vi "Example - Send Client Message.vi"() -> ()   [LabVIEW 2020]
uses:
  <vilib>/ADAS Record/Utilities/TypeDefs/ADAS gRPC/DataStreamGrpc Message.ctl
  <vilib>/ADAS Record/Utilities/ADAS Utilities.lvlib
  <vilib>/DatastreamGrpc/DatastreamGrpc.lvlib
panel:
  in  "Stop":bool
  in  "SEND":bool
  out "error out":errorcluster
  in  "Tab Control":enum32{"Raw JSON", "messageName and Details"}(tab)
  in  "JSON string":string
  in  "messageName":string="Reconfigure"
  in  "details":string="{\"Config Path\":\"C:\\\\Users\\\\Public\\\\Documents\\\\National Instruments\\\\ADAS\\\\Config\\\\test_configB.json\",\"Engine History Length\":1}"
  out "Console Topic Response":string
  in  "timeout (ms)":u32=2000
  in  "Target Topic":T1(ring)
  # "Pre-formatted Reconfigure Details JSON"
  # "{\"Config Path\":\"C:\\\\Users\\\\Public\\\\Documents\\\\National Instruments\\\\ADAS\\\\Config\\\\test_configB.json\",\"Engine History Length\":1}"
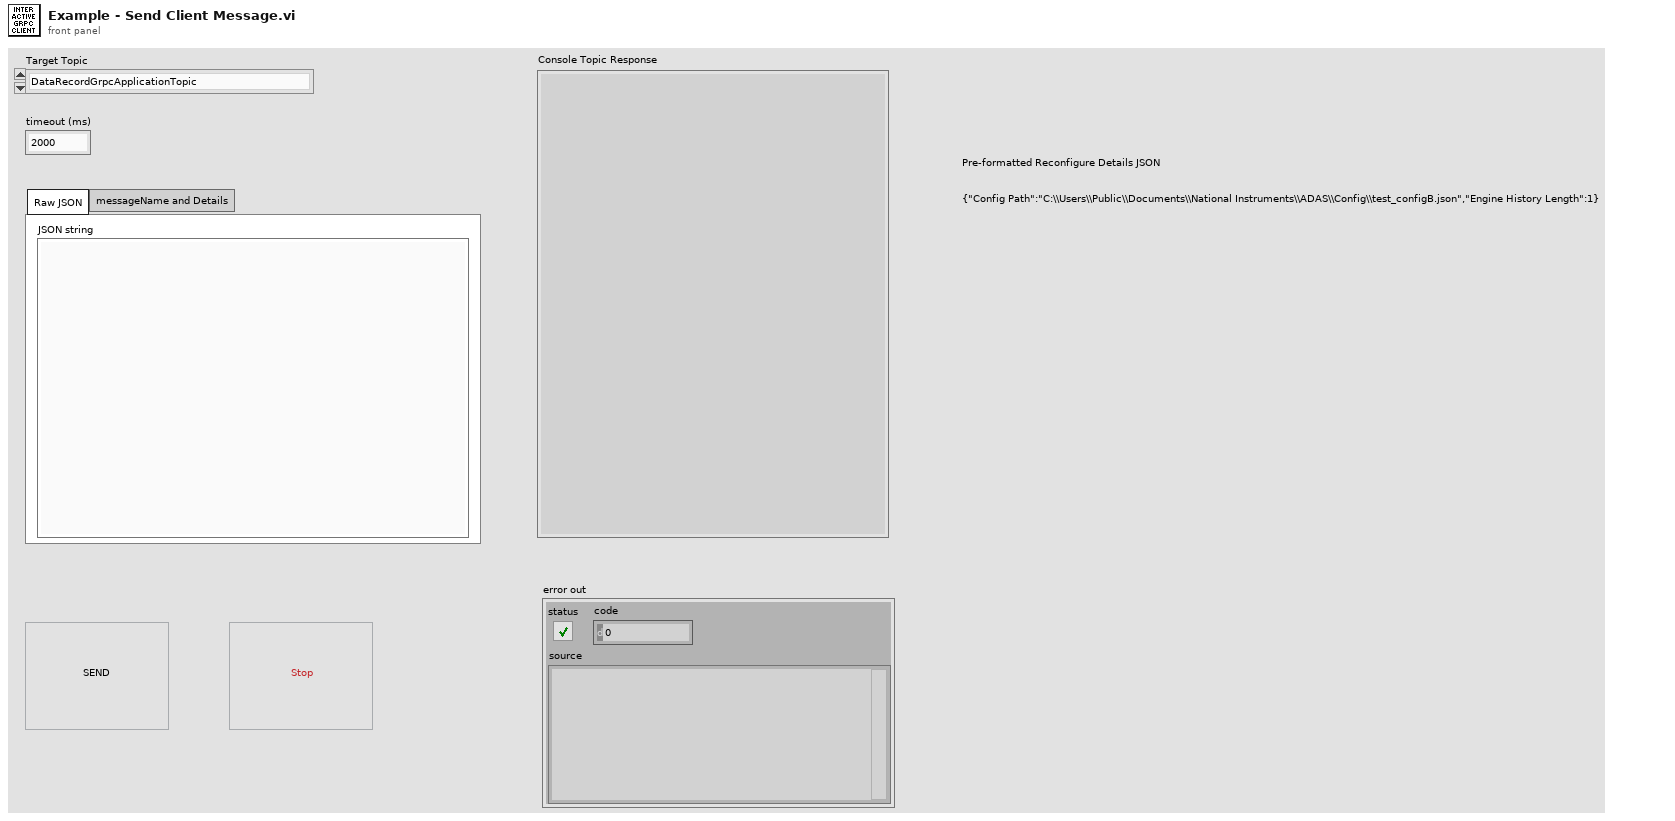
[diagram p1: front panel]
types:
  T1 = enum16{"DataRecordGrpcApplicationTopic", "DataRecordGrpcPluginTopic"}
  T2 = typedef "ADAS Utilities.lvlib/DataStreamGrpc Message.ctl" = cluster{"messageName":string, "details":string}
  T3 = typedef "DatastreamGrpc.lvlib/ClientRef.ctl" = cluster{"id":u64}
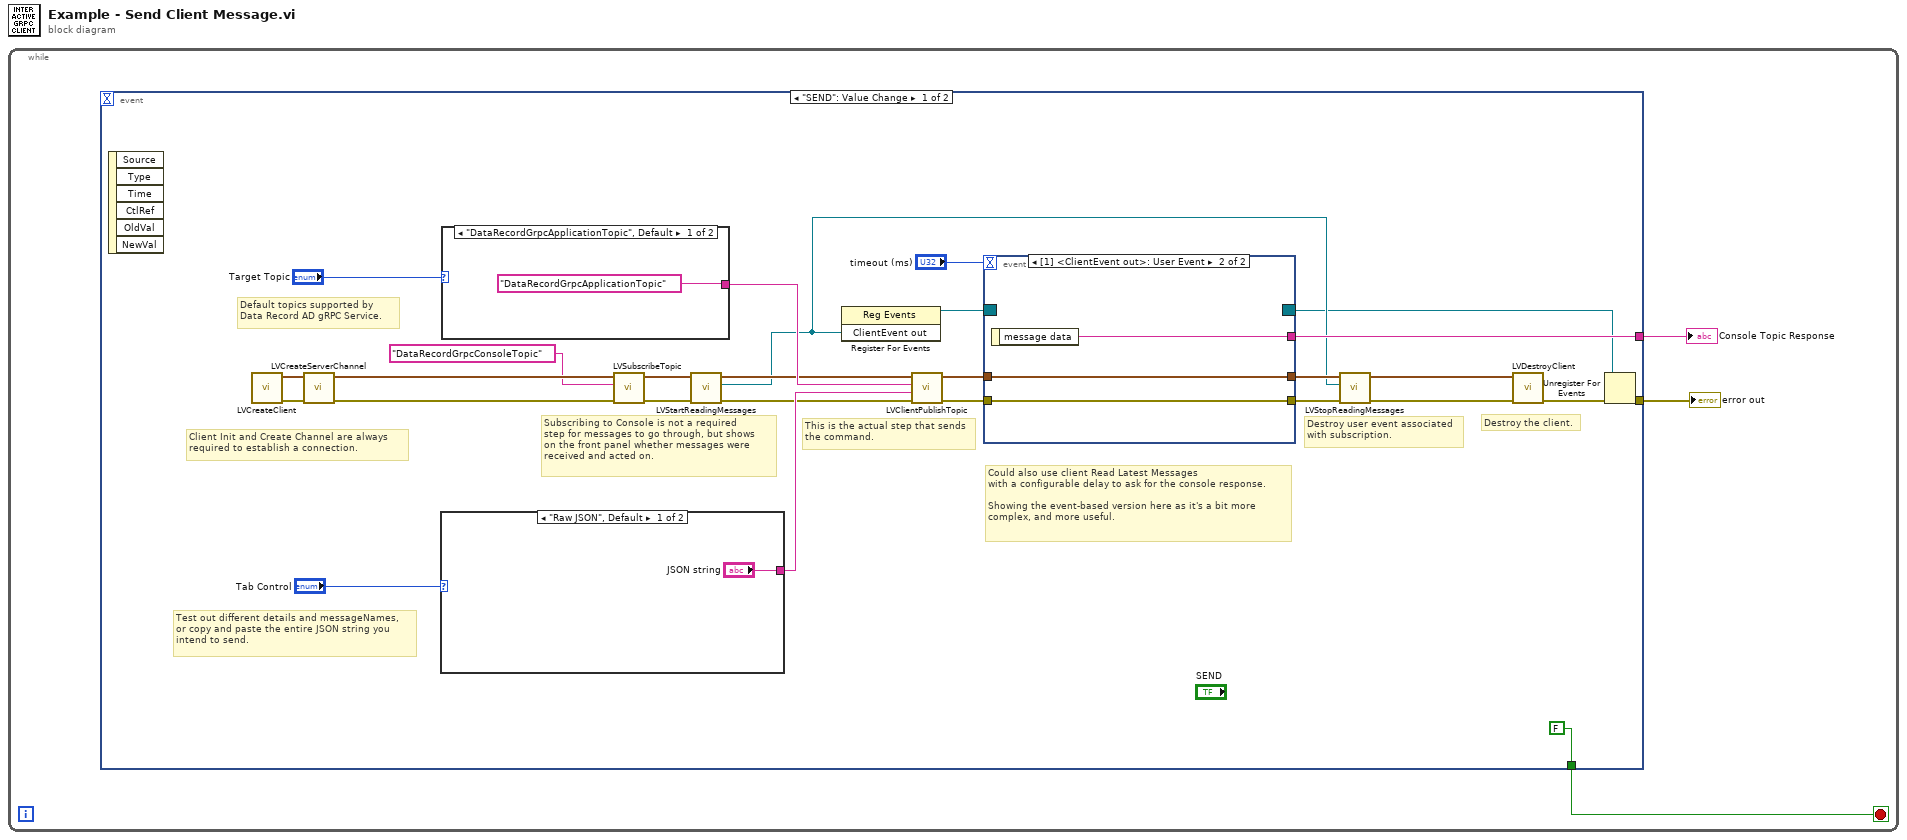
[diagram p0: block diagram]
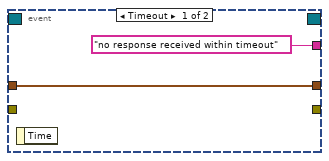
[diagram p2: hidden frame]
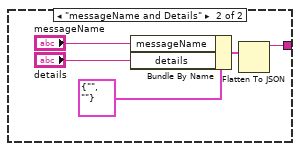
[diagram p3: hidden frame]
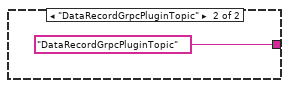
[diagram p4: hidden frame]
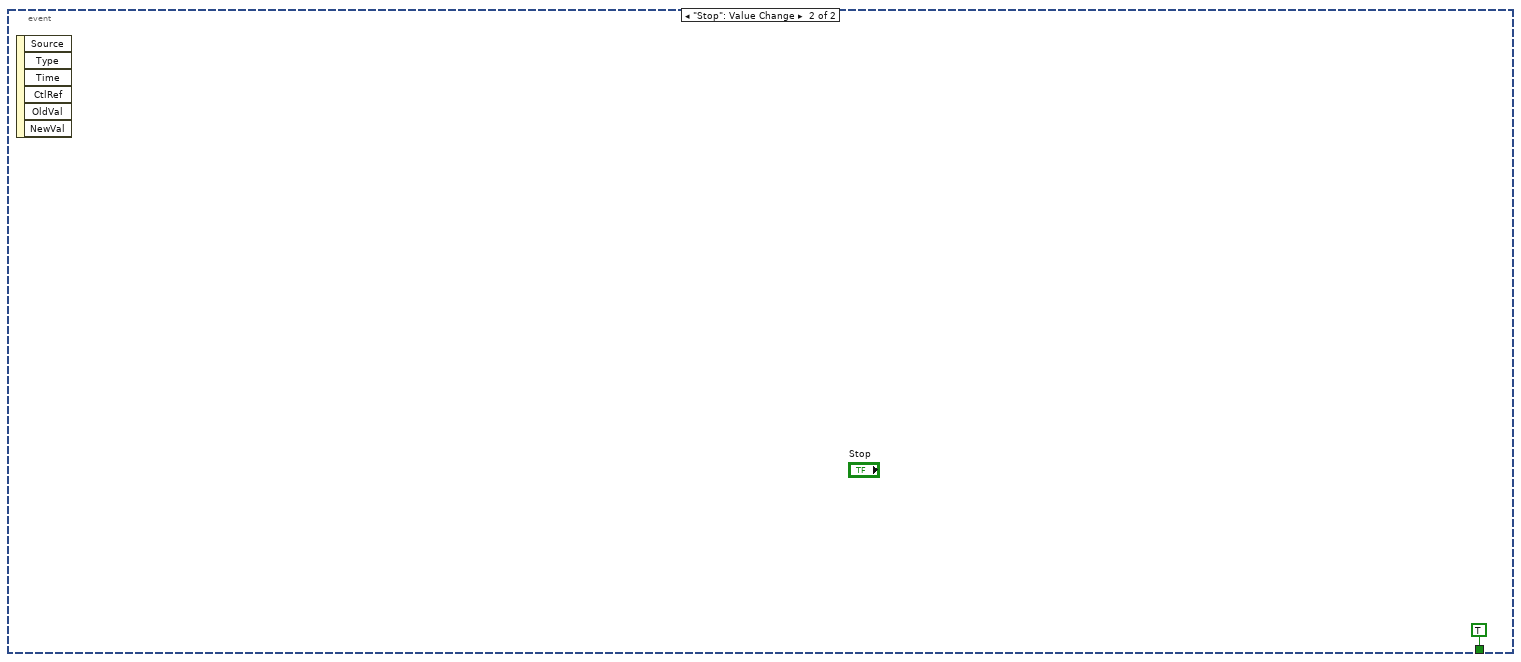
[diagram p5: hidden frame]
diagram:
  n1 = while {
    stop <- w1 stop-if-true
    n2 = event shown="[0] \"SEND\": Value Change" {
      selector: _ -> [_ _]
      dyn-events: _ -> [_ _]
      timeout: _ -> [_ _]
      tunnel: [w15 _] -> w3
      tunnel: [w6 _] -> w2
      tunnel: [FALSE TRUE] -> w1
      event "SEND": Value Change {
        # "Destroy the client."
        # "Destroy user event associated\nwith subscription."
        # "Could also use client Read Latest Messages\nwith a configurable delay to ask for the console response.\n\nShowing the event-based version here as it's a bit more\ncomplex, and more useful."
        # "This is the actual step that sends\nthe command."
        # "Subscribing to Console is not a required \nstep for messages to go through, but shows\non the front panel whether messages were\nreceived and acted on."
        # "Client Init and Create Channel are always \nrequired to establish a connection."
        # "Default topics supported by\nData Record AD gRPC Service."
        # "Test out different details and messageNames,\nor copy and paste the entire JSON string you \nintend to send."
        n3 = event-data() -> ()  [unwired: 1 in, 6 out]
        n4 = call <vilib>:"LVCreateClient.vi"() -> ("error out"=w29:errorcluster, "ClientRef"=w30:T3)  [unwired: 10 in]
        n5 = call <vilib>:"LVCreateServerChannel.vi"("error in (no error)"=w29, "ClientRef in"=w30) -> ("error out"=w27:errorcluster, "ClientRef out"=w28:T3)  [unwired: 8 in]
        n6 = case shown="\"Raw JSON\", Default" "Tab Control" {
          tunnel: ["JSON string" w38] -> w26
          frame "Raw JSON", Default {
          }
          frame "messageName and Details" {
            n7 = Bundle By Name(cluster=T2 {"messageName"="", "details"=""} ("DataStreamGrpc Message"), "messageName"="messageName", "details"="details") -> (w39:T2)
            n8 = Flatten To JSON(anything=w39) -> (JSON string=w38:string)  [unwired: 2 in, 1 out]
          }
        }
        n9 = case shown="\"DataRecordGrpcApplicationTopic\", Default" "Target Topic" {
          tunnel: ["DataRecordGrpcApplicationTopic" "DataRecordGrpcPluginTopic"] -> w24
          frame "DataRecordGrpcApplicationTopic", Default {
          }
          frame "DataRecordGrpcPluginTopic" {
          }
        }
        n10 = call <vilib>:"LVSubscribeTopic.vi"("error in (no error)"=w27, "Topic to subscribe"="DataRecordGrpcConsoleTopic", "ClientRef in"=w28) -> ("error out"=w21:errorcluster, "ClientRef out"=w19:T3)  [unwired: 7 in]
        n11 = call <vilib>:"LVStartReadingMessages.vi"("error in (no error)"=w21, "ClientRef in"=w19) -> ("error out"=w20:errorcluster, "ClientEvent out"=w10:refnum<user-event>, "ClientRef out"=w18:T3)  [unwired: 7 in]
        n12 = register-events(w10) -> (reference out=w16:refnum<event-registration>)  [unwired: 2 in, 1 out]
        n13 = call <vilib>:"LVClientPublishTopic.vi"("error in (no error)"=w20, "MessageData"=w26, "TopicName"=w24, "ClientRef in"=w18) -> ("error out"=w13:errorcluster, "ClientRef out"=w14:T3)  [unwired: 6 in]
        n14 = event shown="[1] <ClientEvent out>: User Event" {
          selector: w16 -> [_ _]
          dyn-events: [_ _] -> w5
          timeout: "timeout (ms)" -> [_ _]
          tunnel: ["no response received within timeout" ("Console Topic Response") w35] -> w15
          tunnel: w14 -> [w31 w34]
          tunnel: [w31 w34] -> w12
          tunnel: [_ w33] -> w9
          tunnel: w13 -> [_ w33]
          event Timeout {
            n15 = event-data() -> ()  [unwired: 1 in, 1 out]
          }
          event User Event {
            n16 = event-data() -> ("message data"=w35:string)  [unwired: 1 in]
          }
        }
        n17 = call <vilib>:"LVStopReadingMessages.vi"("error in (no error)"=w9, "ClientEvent in"=w10, "ClientRef in"=w12) -> ("error out"=w8:errorcluster, "ClientRef out"=w11:T3)  [unwired: 7 in]
        n18 = call <vilib>:"LVDestroyClient.vi"("error in (no error)"=w8, "ClientRef"=w11) -> ("error out"=w7:errorcluster)  [unwired: 9 in]
        n19 = Unregister For Events(event registration refnum=w5, error in=w7) -> (error out=w6:errorcluster)
      }
      event "Stop": Value Change {
        n20 = event-data() -> ()  [unwired: 1 in, 6 out]
      }
    }
    "Console Topic Response" <- w3
    "error out" <- w2
  }
